vi "RateScanAdders_Javi.vi"(0 "ftHandle_in":u32, 5 "VISA resource name":refnum<visa-resource-name>="USB0::0x0957::0x4108::MY51400415::INSTR", 7 "Path":path, 9 "String":string, 11 "error in (no error)":errorcluster) -> (4 "ftHandle_out":u32, 6 "VISA resource name out":refnum<visa-resource-name>, 15 "error out":errorcluster)   [LabVIEW 2019]
uses:
  Global_STOP.vi
panel:
  out "EJECUTANDO TEST SUMADORES":u8(slide) scale=0.0..10.0
  out "Flag_programoPulso":bool
  out "spreadsheet string":string
  out "TOTAL VALORES LLTHX":dbl[][](array[numeric])
  out "Array":u16[](array[numeric])
  out "x*y":u32
  out "TOTAL VALORES HLTHX":dbl[][](array[numeric])
  out "Valor Asic":u16 format="%x"
  out "TOTAL VALORES":u16[][](array[numeric]) format="%x"
  out "DAC TH3,TH4,TH5":u16
  out "LLTHx":dbl
  out "DAC TH0,TH1,TH2":u16
  out "HLTHx":dbl
  # "IN"
  # "1 + 2 + 3"
  # "ADC"
  # "ADC"
  # "Vin Asic"
  # "Vin Asic"
  # "ADD A/1"
  # "ADD B/1"
  # "ADD C/1"
  # "ADD A/0"
  # "ADD B/0"
  # "ADD C/0"
  # "50mV"
  # "50mV"
  # "90mV"
  # "90mV"
  # "130mV"
  # "130mV"
  # "170mV"
  # "170mV"
  # "210mV"
  # "210mV"
  # "250mV"
  # "250mV"
  # "290mV"
  # "290mV"
  # "330mV"
  # "330mV"
  # "370mV"
  # "370mV"
  # "410mV"
  # "410mV"
  # "TH0"
  # "TH1"
  # "TH2"
  # "DAC"
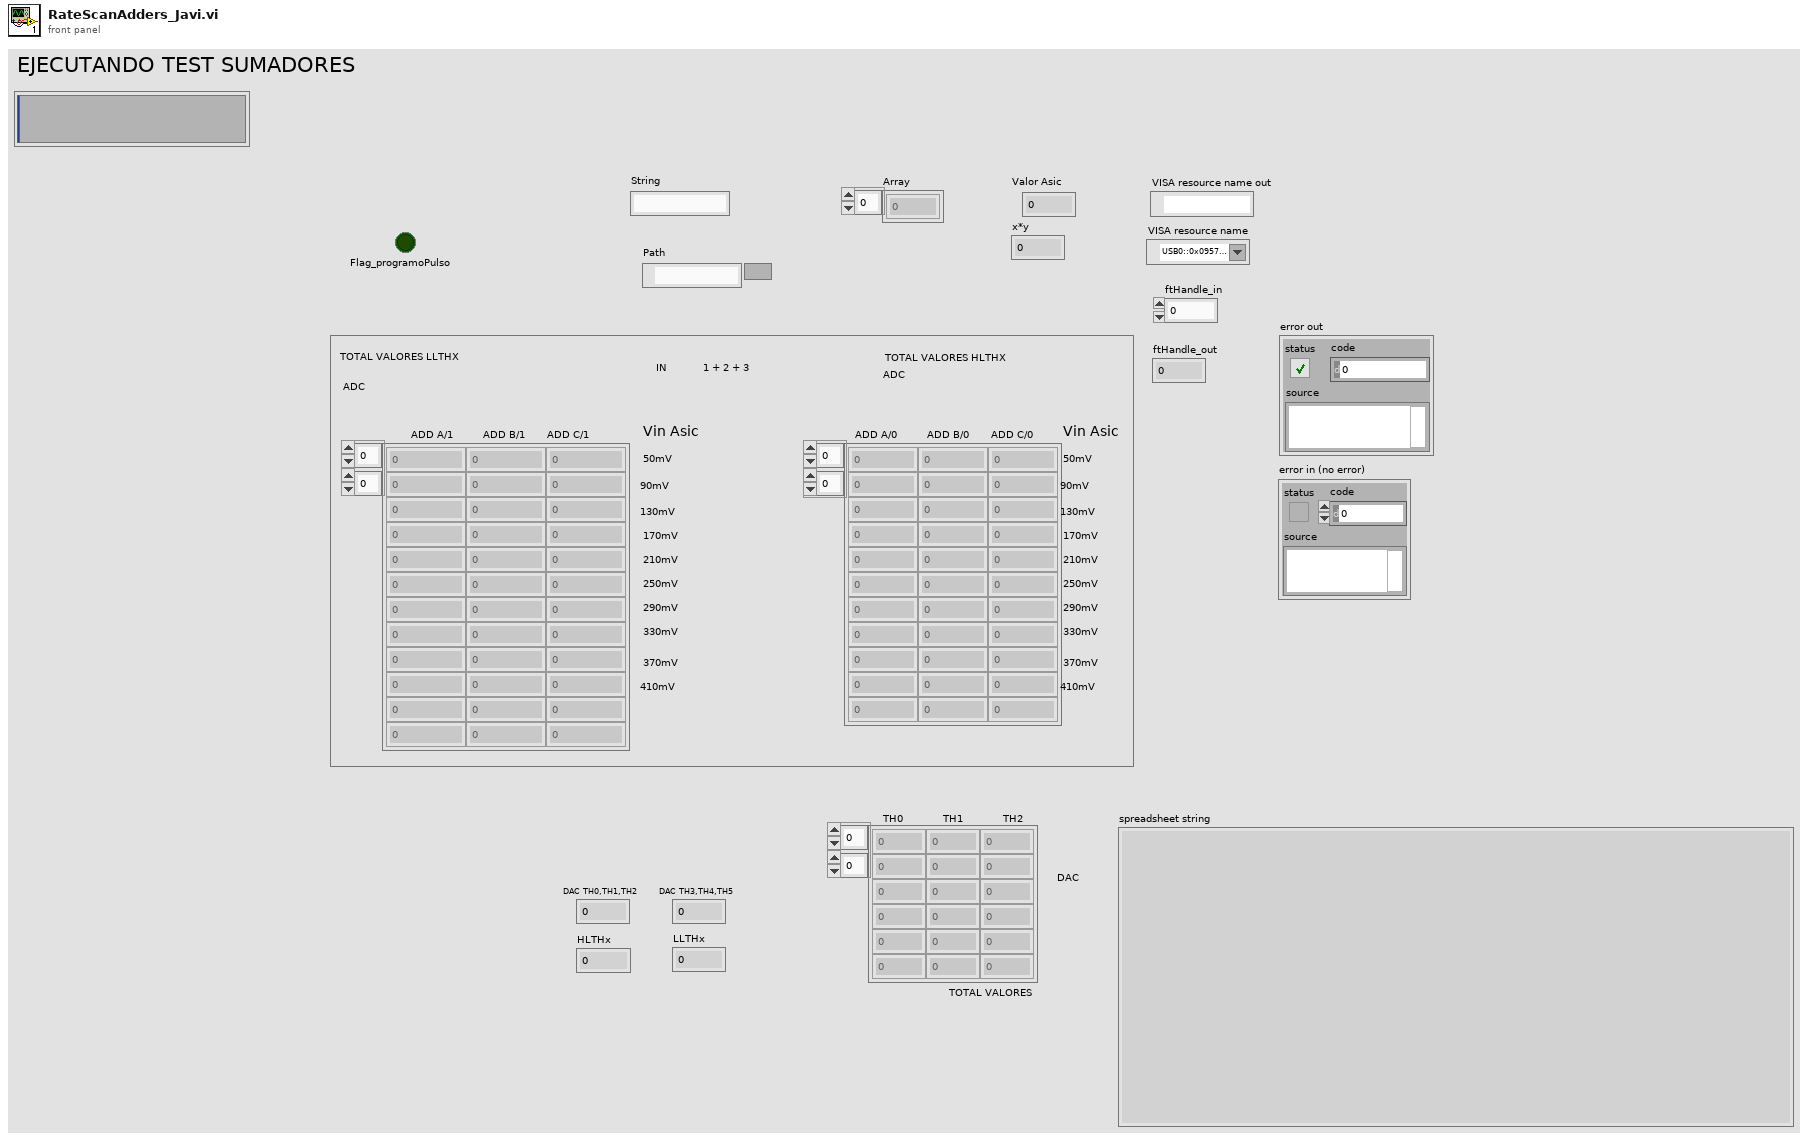
[diagram p1: front panel]
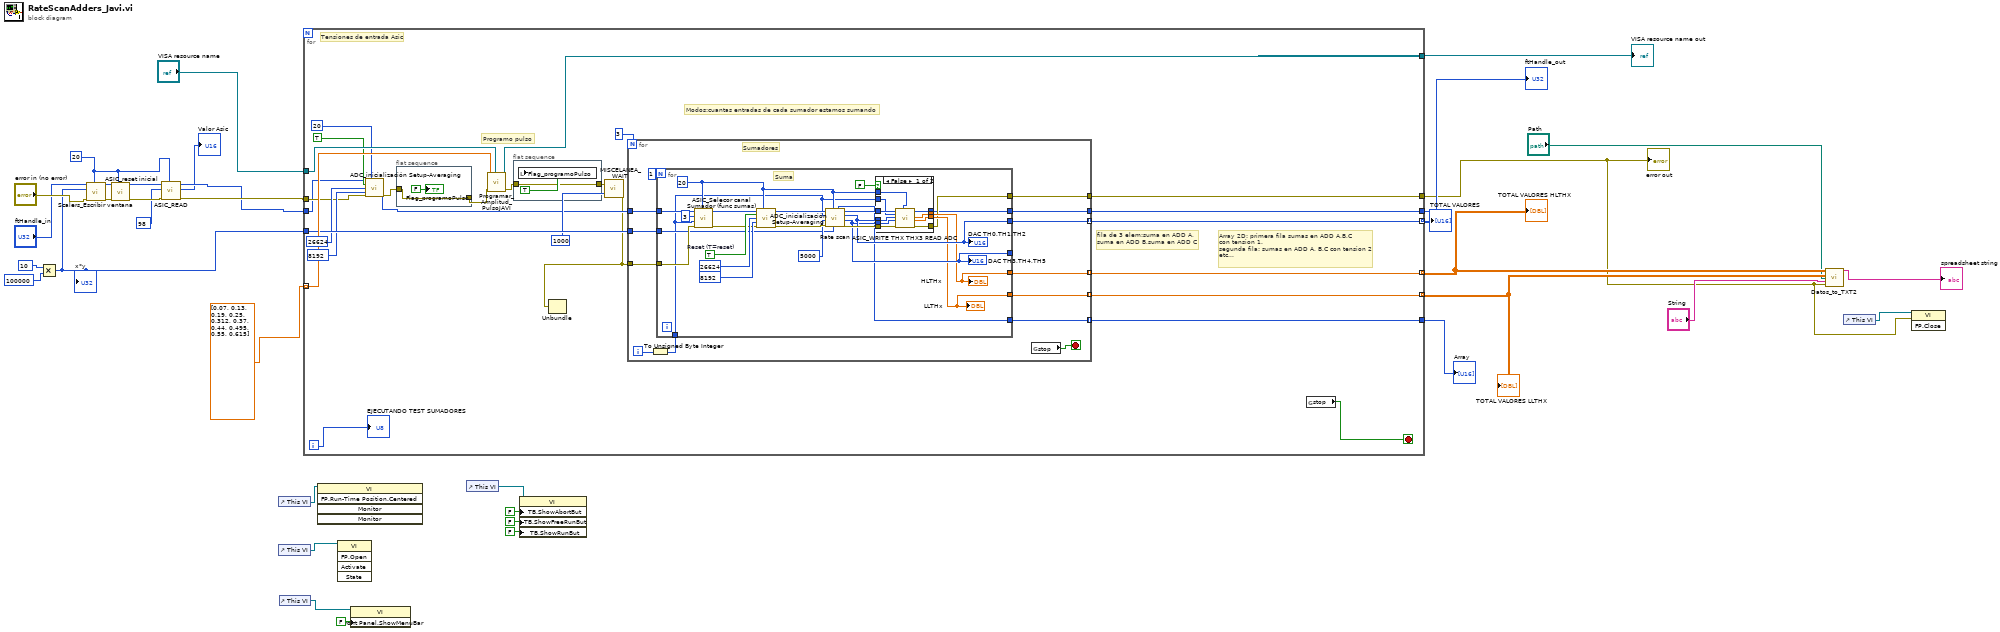
[diagram p0: block diagram]
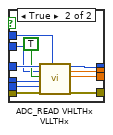
[diagram p2: hidden frame]
diagram:
  w18 = u32 20 ("Espera acceso USB")
  n1 = Multiply(x=u32 10 ("Ventana"), y=u32 100000 ("Ventana")) -> (x*y=w28:u32)
  "x*y" <- w28
  n2 = call "Scalers_Escribir ventana.vi"("Espera acceso USB"=w18, "error in"="error in (no error)", "Ventana"=w28, "ftHandle_in"="ftHandle_in") -> ("error out"=w33:errorcluster, "ftHandle_out"=w32:u32)  [unwired: 6 in]
  n3 = call "ASIC_reset inicial.vi"("Espera acceso USB"=w18, "error in"=w33, "ftHandle_in"=w32) -> ("error out"=w23:errorcluster, "ftHandle_out"=w24:u32)  [unwired: 7 in]
  n4 = call "ASIC_READ.vi"("Espera acceso USB"=w18, "error in"=w23, "Direccion Registro Asic"=u8 98, "ftHandle_in"=w24) -> ("error out"=w22:errorcluster, "Valor Asic"=→"Valor Asic":u16, "ftHandle_out"=w21:u32)  [unwired: 5 in]
  n5 = control-ref of="This VI"() -> (w10:refnum<vi>)
  n6 = control-ref of="This VI"() -> (w7:refnum<vi>)
  n7 = control-ref of="This VI"() -> (w6:refnum<vi>)
  n8 = for {
    tunnel: dbl[] [0.07, 0.13, 0.19, 0.25, 0.312, 0.37, 0.44, 0.495, 0.55, 0.615] -> [w61] mode=indexing
    tunnel: "VISA resource name" -> [w60]
    tunnel: w21 -> [w47]
    tunnel: w22 -> [w49]
    tunnel: w28 -> [w59]
    tunnel: [w58] -> w8
    tunnel: [w57] -> w27
    tunnel: [w56] -> w26
    tunnel: [w55] -> w25 mode=indexing
    tunnel: [w54] -> w17
    tunnel: [w44] -> w15 mode=indexing
    tunnel: [w43] -> w14 mode=indexing
    i -> [w36]
    stop <- w37 stop-if-true
    # "fila de 3 elem:suma en ADD A,\nsuma en ADD B,suma en ADD C"
    # "Modos:cuantas entradas de cada sumador estamos sumando"
    # "Array 2D: primera fila sumas en ADD A,B,C\ncon tension 1.\nsegunda fila: sumas en ADD A, B,C con tension 2\netc..."
    # "Programo pulso"
    # "Tensiones de entrada Asic"
    n9 = call "ADC_inicialización Setup-Averaging.vi"("ftHandle_in 2"=w47, "Espera acceso USB"=u32 20, "Reset (T=reset)"=TRUE, "Registro Setup (0x6800)"=u16 26624, "Registro Averaging (0x3200)"=u16 8192 ("Registro Setup (0x6800)"), "error in 2"=w49) -> ("ftHandle_out"=w46:u32, "error out"=w41:errorcluster)  [unwired: 8 in]
    n10 = flat-sequence {
      tunnel: [w65] -> w40
      tunnel: w41 -> [w65]
      frame #0 {
        "Flag_programoPulso" <- FALSE ("Flag_programoPulso")
      }
    }
    n11 = call "Programar_Amplitud_PulsoJAVI.vi"("error in (no error)"=w40, "Numeric"=w61, "VISA Refnum in"=w60) -> ("Error OUT"=w39:errorcluster, "VISA resource name out"=w57:refnum<visa-resource-name>)  [unwired: 7 in]
    n12 = flat-sequence {
      tunnel: w39 -> [w62]
      tunnel: [w62] -> w38
      frame #0 {
        n13 = local write "Flag_programoPulso"(TRUE ("Flag_programoPulso")) -> ()
      }
    }
    n14 = call "MISCELANEA_WAIT.vi"("ms wait IN"=u32 1000, "Error IN"=w38) -> ("Error OUT"=w42:errorcluster)  [unwired: 16 in, 1 out]
    n15 = Unbundle(w42) -> ()  [unwired: 3 out]
    n16 = for {
      N: 3 -> [_]
      tunnel: w46 -> [w77]
      tunnel: w42 -> [w74]
      tunnel: w59 -> [w73]
      tunnel: [w72] -> w55 mode=indexing
      tunnel: [w71] -> w58
      tunnel: [w70] -> w56
      tunnel: [w69] -> w54 mode=indexing
      tunnel: [w68] -> w44 mode=indexing
      tunnel: [w67] -> w43 mode=indexing
      i -> [w76]
      stop <- w66 stop-if-true
      # "Sumadores"
      n17 = To Unsigned Byte Integer(number=w76) -> (unsigned 8bit integer=w75:u8)
      n18 = for {
        N: 1 -> [_]
        tunnel: w77 -> [w91]
        tunnel: w75 -> [w80]
        tunnel: w74 -> [w90]
        tunnel: w73 -> [w88]
        tunnel: [w87] -> w72
        tunnel: [w86] -> _
        tunnel: [w85] -> w68
        tunnel: [w84] -> w67
        tunnel: [w83] -> w71
        tunnel: [w82] -> w69
        tunnel: [w81] -> w70
        w89 = u32 20 ("Espera acceso USB")
        w102 = TRUE  # Reset (T=reset)
        # "Suma"
        n19 = call "ASIC_Selecor canal Sumador (func sumas).vi"("Espera acceso USB"=w89, "error in"=w90, "Sumador"=w80, "Modo"=u8 3, "ftHandle_in"=w91) -> ("error out"=w97:errorcluster, "ftHandle_out"=w94:u32)  [unwired: 3 in, 2 out]
        n20 = call "ADC_inicialización Setup-Averaging.vi"("ftHandle_in 2"=w94, "Espera acceso USB"=w89, "Reset (T=reset)"=w102, "Registro Setup (0x6800)"=u16 26624, "Registro Averaging (0x3200)"=u16 8192 ("Registro Setup (0x6800)"), "error in 2"=w97) -> ("ftHandle_out"=w99:u32, "error out"=w98:errorcluster)  [unwired: 8 in]
        n21 = call "Rate scan.vi"("T Ventana"=w88, "Espera acceso USB"=w89, "error in 2"=w98, "Valor buscado scalers (5000)"=u16 5000 ("Valor buscado scalers"), "Sumador"=w80, "ftHandle_in 2"=w99) -> ("error out 2"=w95:errorcluster, "DAC\nTH3,TH4,TH5"=w86:u16, "DAC\nTH0,TH1,TH2"=w87:u16, "ftHandle_out 2"=w96:u32, "Scaler 1"=w82:u16)  [unwired: 1 in]
        "DAC TH0,TH1,TH2" <- w87
        "DAC TH3,TH4,TH5" <- w86
        n22 = case shown="False" FALSE {
          tunnel: w96 -> [w112 w123]
          tunnel: w95 -> [w109 w122]
          tunnel: [w107 w121] -> w81
          tunnel: [w108 w120] -> w83
          tunnel: [w106 w119] -> w85
          tunnel: [w105 w118] -> w84
          tunnel: w87 -> [w111 w117]
          tunnel: w86 -> [w110 w116]
          tunnel: w89 -> [w104 w114]
          tunnel: w80 -> [w103 w113]
          frame False {
            n23 = call "ASIC_WRITE THX THX3 READ ADC.vi"("ftHandle_in"=w112, "Sumador"=w103, "THX"=w111, "THX+3"=w110, "error in"=w109, "Espera acceso USB 2"=w104) -> ("ftHandle_out"=w107:u32, "HLTHx"=w106:dbl, "LLTHx"=w105:dbl, "error out"=w108:errorcluster)  [unwired: 10 in]
          }
          frame True {
            n24 = call "ADC_READ VHLTHx VLLTHx.vi"("ftHandle_out 2"=w123, "Sumador"=w113, "referenciar"=TRUE, "ref DAC\nTH0,TH1,TH2"=w117, "ref DAC\nTH3,TH4,TH5"=w116, "error out 2"=w122, "Espera acceso FT"=w114) -> ("ftHandle_out"=w121:u32, "HLTHx"=w119:dbl, "LLTHx"=w118:dbl, "error out"=w120:errorcluster)  [unwired: 8 in, 1 out]
          }
        }
        "HLTHx" <- w85
        "LLTHx" <- w84
      }
      n25 = global read "Global_STOP.vi" "stop"() -> (w66:bool)
    }
    n26 = global read "Global_STOP.vi" "stop"() -> (w37:bool)
    "EJECUTANDO TEST SUMADORES" <- w36
  }
  "error out" <- w8
  "VISA resource name out" <- w27
  "ftHandle_out" <- w26
  "TOTAL VALORES" <- w25
  "TOTAL VALORES HLTHX" <- w15
  "Array" <- w17
  "TOTAL VALORES LLTHX" <- w14
  n27 = invoke class="VI" method="FP.Run-Time Position.Centered"(reference=w10) -> ()  [unwired: 4 in, 5 out]
  n28 = invoke class="VI" method="FP.Open"(reference=w7) -> ()  [unwired: 4 in, 5 out]
  n29 = property class="VI"(reference=w6, "Front Panel.ShowMenuBar"=FALSE ("Front Panel Window:Show Menu Bar")) -> ()  [unwired: 1 in, 2 out]
  n30 = control-ref of="This VI"() -> (w4:refnum<vi>)
  n31 = property class="VI"(reference=w4, "TB.ShowAbortBut"=FALSE ("Tool Bar:Show Abort Button"), "TB.ShowFreeRunBut"=FALSE ("Tool Bar:Show Free Run Button"), "TB.ShowRunBut"=FALSE ("Tool Bar:Show Run Button")) -> ()  [unwired: 1 in, 2 out]
  n32 = call "Datos_to_TXT2.vi"("Array"=w15, "Array 2"=w14, "Path"="Path", "String"="String", "error in (no error)"=w8) -> ("spreadsheet string"=→"spreadsheet string":string)  [unwired: 10 in]
  n33 = control-ref of="This VI"() -> (w9:refnum<vi>)
  n34 = invoke class="VI" method="FP.Close"(reference=w9, error in=w8) -> ()  [unwired: 1 in, 3 out]
